vi "Modbus Status Interface.vi"(0 "ES System Data In":T8={"Voltage"=0.0, "Current"=0.0, "SOC Avg"=0.0, "Faults"=0, "Alarms"=0, "# Strings"=0, "Max Temp"=0, "Min Temp"=0, "Max Cell Voltage"=0.0, "Min Cell Voltage"=0.0, "Energy Capacity"=0.0, "Energy Remaining"=0.0, "SOC Min"=0.0, "SOC Max"=0.0, "ES Fault"=FALSE, "String Select"=enum."3 Strings", "ES Com Fault"=FALSE, "SOH Avg"=0.0}, 1 "ES String Data":T2, 2 "Gen Data Array":T4[](array[typedef]) {"TotalFuel(L)" format="%.2f"; "FuelRate(L/H)" format="%.2f"; "ApparentPower(VA)" format="%.2f"; "BattVoltage(V)" format="%.2f"; "Freq(Hz)" format="%.2f"; "RunHours(hr)" format="%.2f"; "PowerFactor" format="%.2f"; "ReactivePower(VAR)" format="%.2f"; "ActivePower(W)" format="%.2f"}, 3 "ES # Cycle Count":dbl, 5 "PC Data In":T6 {"Alarms 2" format="%016b"; "Faults 2" format="%016b"; "Alarms 1" format="%016b"; "Faults 1" format="%016b"; "Contactor FB" format="%.0b"; "DC Voltage SP" format="%2.1f"; "Clear Faults SP" format="%.0b"; "Neutral Current" format="%2.1f"; "AC Current - L2" format="%2.1f"; "AC Voltage - L2" format="%2.1f"; "Temperature" format="%2.1f"; "DC Voltage" format="%2.1f"; "AC Current SP" format="%2.1f"; "AC Voltage SP" format="%2.1f"; "Frequency SP" format="%2.1f"; "AC Frequency" format="%2.1f"; "AC Current - L1" format="%2.1f"; "AC Voltage- L1" format="%2.1f"}, 7 "isGenOn":bool[](array[boolean]), 9 "FPGA Data In":T5 {"SSG Active Current" format="%2.1f"; "PV Reactive Power (L1)" format="%2.1f"; "PV Reactive Power (L2)" format="%2.1f"; "PV Total Reactive Power" format="%2.1f"; "Gen Reactive Power (L1)" format="%2.1f"; "Gen Reactive Power (L2)" format="%2.1f"; "Gen Total Reactive Power" format="%2.1f"; "SSG Reactive Power (L1)" format="%2.1f"; "SSG Reactive Power (L2)" format="%2.1f"; "SSG Total Reactive Power" format="%2.1f"; "PV Total Current" format="%2.1f"; "PV Total Voltage" format="%2.1f"; "PV Active Power (L1)" format="%2.1f"; "PV Active Power (L2)" format="%2.1f"; "PV App Power (L1)" format="%2.1f"; "PV App Power (L2)" format="%2.1f"; "PV Total Active Power" format="%2.1f"; "PV Total App Power" format="%2.1f"; "PV Arms (L1)" format="%2.1f"; "PV Arms (L2)" format="%2.1f"; "PV Vrms (L1)" format="%2.1f"; "PV Vrms (L2)" format="%2.1f"; "Gen Total Current" format="%2.1f"; "SSG Total Current" format="%2.1f"; "Gen Total Voltage" format="%2.1f"; "SSG Total Voltage" format="%2.1f"; "Gen Active Power (L1)" format="%2.1f"; "Gen Active Power (L2)" format="%2.1f"; "SSG Active Power (L1)" format="%2.1f"; "SSG Active Power (L2)" format="%2.1f"; "Gen App Power (L1)" format="%2.1f"; "Gen App Power (L2)" format="%2.1f"; "SSG App Power (L1)" format="%2.1f"; "SSG App Power (L2)" format="%2.1f"; "Gen Total Active Power" format="%2.1f"; "Gen Total App Power" format="%2.1f"; "Gen Arms (L1)" format="%2.1f"; "Gen Arms (L2)" format="%2.1f"; "Gen Vrms (L1)" format="%2.1f"; "Gen Vrms (L2)" format="%2.1f"; "SSG Total Active Power" format="%2.1f"; "SSG Total App Power" format="%2.1f"; "SSG Arms (L1)" format="%2.1f"; "SSG Arms (L2)" format="%2.1f"; "SSG Vrms (L1)" format="%2.1f"; "SSG Vrms (L2)" format="%2.1f"}, 11 "Error In":errorcluster, 12 "Real Time State":T1) -> (15 "Error Out":errorcluster)   [LabVIEW 2014]
uses:
  Controls/ES System Data.ctl
  Controls/StringSelector.ctl
  Controls/PC Data.ctl
  Controls/MicroZed Config Op Mode.ctl
  Controls/FPGA Data.ctl
  Controls/Gen Data.ctl
  Controls/ES String Array.ctl
  Controls/ES String Data.ctl
  Controls/RT State.ctl
  Controls/Interface Data.ctl
panel:
  # "West"
  # "East"
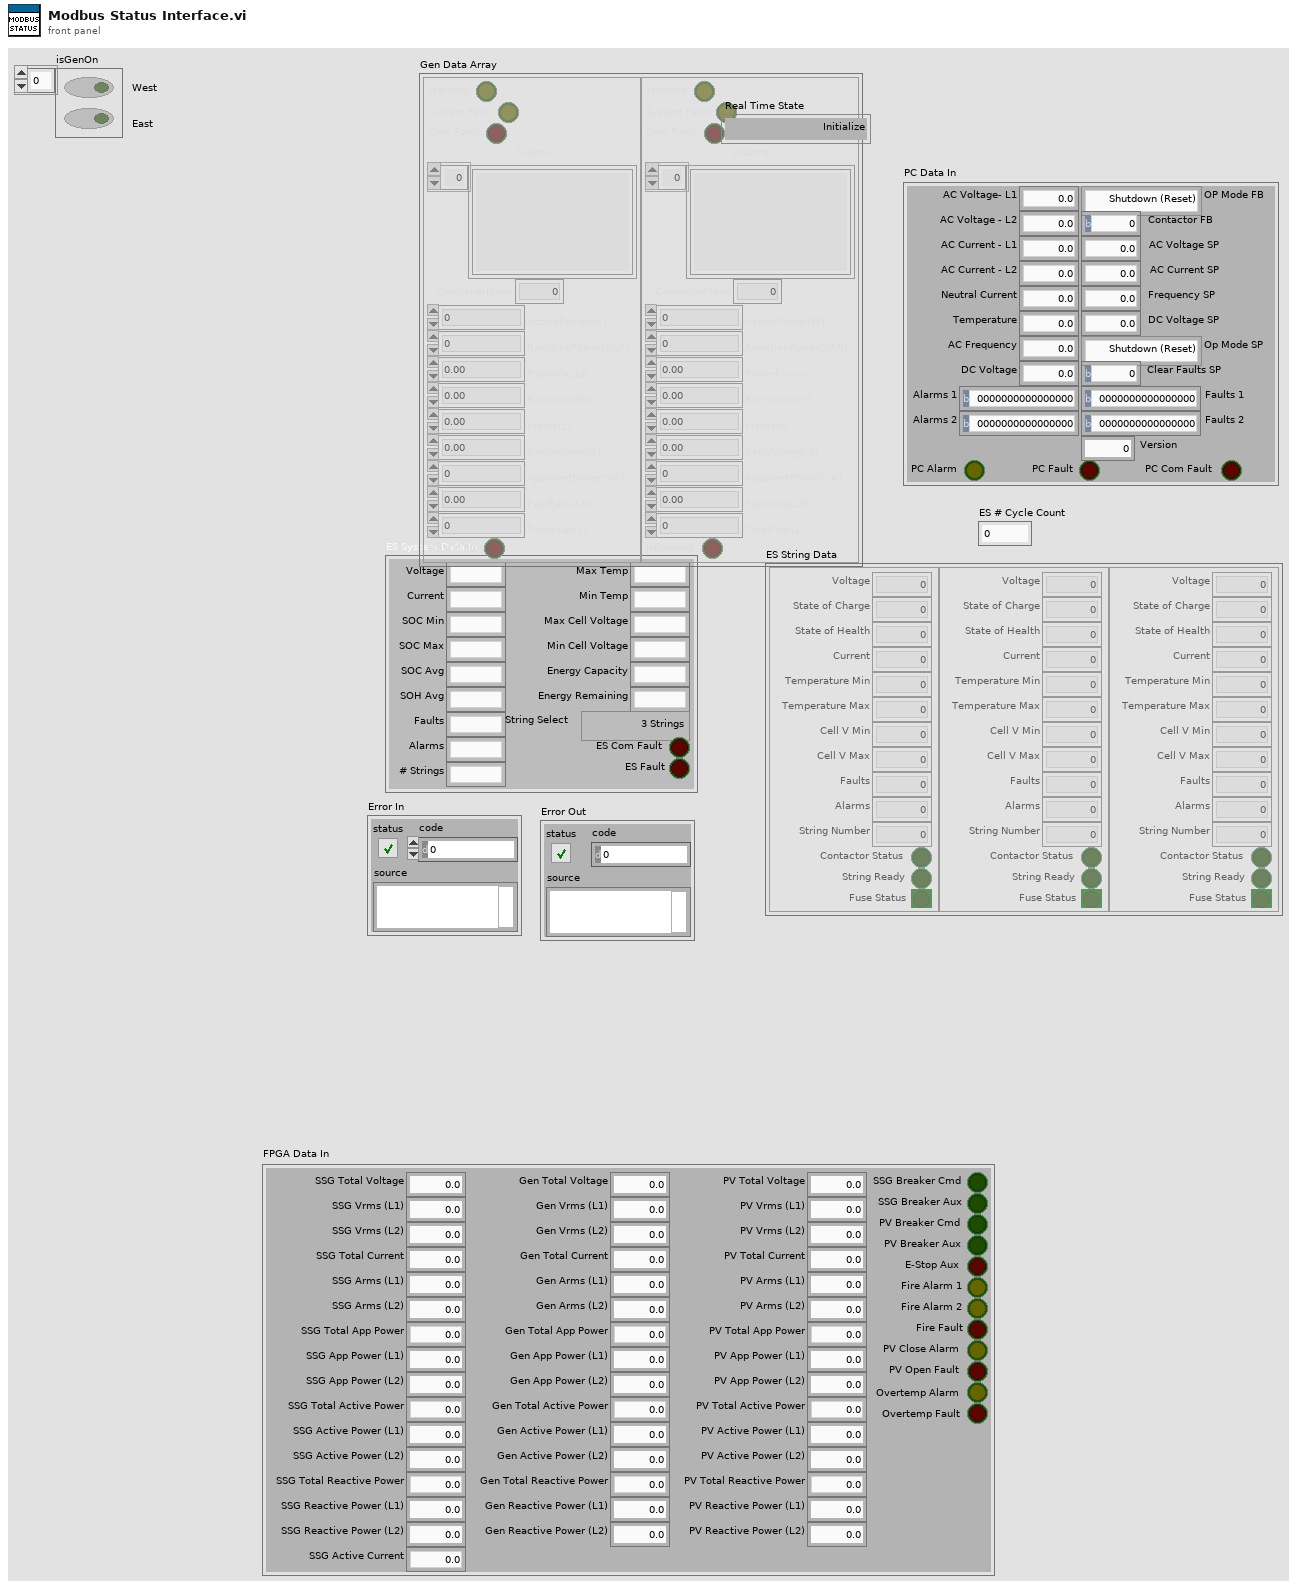
[diagram p1: front panel]
types:
  T1 = typedef "RT State.ctl" = enum16{"Initialize", "Ready", "Startup 1 - Start Genset", "Startup 2 - Start Inverter", "Startup 3 - Battery Match", "SpotGen - Start", "SpotGen - Charge", "SpotGen - Desync", "SpotGen - Discharge", "SpotGen - Sync", "Shutdown", "INVALID STATE"}
  T2 = typedef "ES String Array.ctl" = T3[]
  T3 = typedef "ES String Data.ctl" = cluster{"Voltage":sgl, "State of Charge":sgl, "Current":sgl, "Temperature Min":i16, "Temperature Max":i16, "Faults":u16, "Alarms":u16, "String Number":u16, "Contactor Status":bool, "String Ready":bool, "Fuse Status":bool, "Cell V Max":dbl, "Cell V Min":dbl, "State of Health":sgl}
  T4 = typedef "Gen Data.ctl" = cluster{"Warning":bool, "System Fault":bool, "Com Fault":bool, "Alarms":string[], "ControllerMode":u16, "ActivePower(W)":i32, "ReactivePower(VAR)":i32, "PowerFactor":dbl, "RunHours(hr)":dbl, "Freq(Hz)":dbl, "BattVoltage(V)":dbl, "ApparentPower(VA)":i32, "FuelRate(L/H)":dbl, "TotalFuel(L)":u32, "IsRunning":bool}
  T5 = typedef "FPGA Data.ctl" = cluster{"Gen Total Voltage":dbl, "Gen Vrms (L1)":dbl, "Gen Vrms (L2)":dbl, "Gen Total Current":dbl, "Gen Arms (L1)":dbl, "Gen Arms (L2)":dbl, "Gen Total App Power":dbl, "Gen App Power (L1)":dbl, "Gen App Power (L2)":dbl, "Gen Total Active Power":dbl, "Gen Active Power (L1)":dbl, "Gen Active Power (L2)":dbl, "Gen Total Reactive Power":dbl, "Gen Reactive Power (L1)":dbl, "Gen Reactive Power (L2)":dbl, "SSG Total Voltage":dbl, "SSG Vrms (L1)":dbl, "SSG Vrms (L2)":dbl, "SSG Total Current":dbl, "SSG Arms (L1)":dbl, "SSG Arms (L2)":dbl, "SSG Total App Power":dbl, "SSG App Power (L1)":dbl, "SSG App Power (L2)":dbl, "SSG Total Active Power":dbl, "SSG Active Power (L1)":dbl, "SSG Active Power (L2)":dbl, "SSG Total Reactive Power":dbl, "SSG Reactive Power (L1)":dbl, "SSG Reactive Power (L2)":dbl, "PV Total Voltage":dbl, "PV Vrms (L1)":dbl, "PV Vrms (L2)":dbl, "PV Total Current":dbl, "PV Arms (L1)":dbl, "PV Arms (L2)":dbl, "PV Total App Power":dbl, "PV App Power (L1)":dbl, "PV App Power (L2)":dbl, "PV Total Active Power":dbl, "PV Active Power (L1)":dbl, "PV Active Power (L2)":dbl, "PV Total Reactive Power":dbl, "PV Reactive Power (L1)":dbl, "PV Reactive Power (L2)":dbl, "SSG Breaker Cmd":bool, "SSG Breaker Aux":bool, "PV Breaker Cmd":bool, "PV Breaker Aux":bool, "E-Stop Aux":bool, "Fire Alarm 1":bool, "Fire Alarm 2":bool, "Fire Fault":bool, "PV Close Alarm":bool, "SSG Active Current":dbl, "Overtemp Alarm":bool, "Overtemp Fault":bool, "PV Open Fault":bool}
  T6 = typedef "PC Data.ctl" = cluster{"AC Voltage- L1":dbl, "AC Voltage - L2":dbl, "AC Current - L1":dbl, "AC Current - L2":dbl, "Neutral Current":dbl, "Temperature":dbl, "AC Frequency":dbl, "DC Voltage":dbl, "AC Voltage SP":dbl, "AC Current SP":dbl, "Frequency SP":dbl, "Op Mode SP":T7, "Clear Faults SP":u16, "PC Com Fault":bool, "PC Fault":bool, "DC Voltage SP":dbl, "OP Mode FB":T7, "Contactor FB":u16, "Faults 1":u16, "Alarms 1":u16, "Faults 2":u16, "Alarms 2":u16, "PC Alarm":bool, "Version":u16}
  T7 = typedef "MicroZed Config Op Mode.ctl" = enum16{"Shutdown (Reset)", "Startup", "Idle", "Voltage Mode", "Current Mode", "Fault", "OL Voltage (Debug)", "No Data"}
  T8 = typedef "ES System Data.ctl" = cluster{"Voltage":sgl, "Current":sgl, "SOC Avg":sgl, "Faults":u16, "Alarms":u16, "# Strings":u16, "Max Temp":i16, "Min Temp":i16, "Max Cell Voltage":sgl, "Min Cell Voltage":sgl, "Energy Capacity":sgl, "Energy Remaining":sgl, "SOC Min":sgl, "SOC Max":sgl, "ES Fault":bool, "String Select":T9, "ES Com Fault":bool, "SOH Avg":sgl}
  T9 = typedef "StringSelector.ctl" = enum16{"1 String (1)", "1 String (2)", "1 String (3)", "2 Strings (1 2)", "2 Strings (2 3)", "2 Strings (1 3)", "3 Strings"}
  T10 = typedef "Interface Data.ctl" = cluster{"SSG AC Current":i16, "SSG AC Voltage":i16, "SSC Active Power":i16, "SSG Reactive Power":i16, "SSG Apparent Power":i16, "SSG Frequency":i16, "ES SOC":i16, "ES SOH":i16, "ES Voltage":i16, "ES # Strings":i16, "ES # Cycles":i16, "ES Temperature":i16, "PC Temperature":i16, "Solar Active Power":i16, "Converter Version":i16, "Controller Version":i16, "System Status":i16, "System Faults":i16, "Controller Faults":i16, "ES System Faults":i16, "ES System Alarms":i16, "Converter Faults 1":i16, "Converter Faults 2":i16, "Converter Alarms 1":i16, "Converter Alarms 2":i16, "Solar Faults":i16, "ES Rack 1 Faults":i16, "ES Rack 2 Faults":i16, "ES Rack 3 Faults":i16, "ES Rack 4 Faults":i16, "ES Rack 5 Faults":i16, "ES Rack 6 Faults":i16, "ES Rack 7  Faults":i16, "ES Rack 8 Faults":i16, "ES Rack 9 Faults":i16, "ES Rack 10 Faults":i16, "ES Rack 1 Alarms":i16, "ES Rack 2 Alarms":i16, "ES Rack 3 Alarms":i16, "ES Rack 4 Alarms":i16, "ES Rack 5 Alarms":i16, "ES Rack 6 Alarms":i16, "ES Rack 7 Alarms":i16, "ES Rack 8 Alarms":i16, "ES Rack 9 Alarms":i16, "ES Rack 10 Alarms":i16, "GenWest":T4, "GenEast":T4}
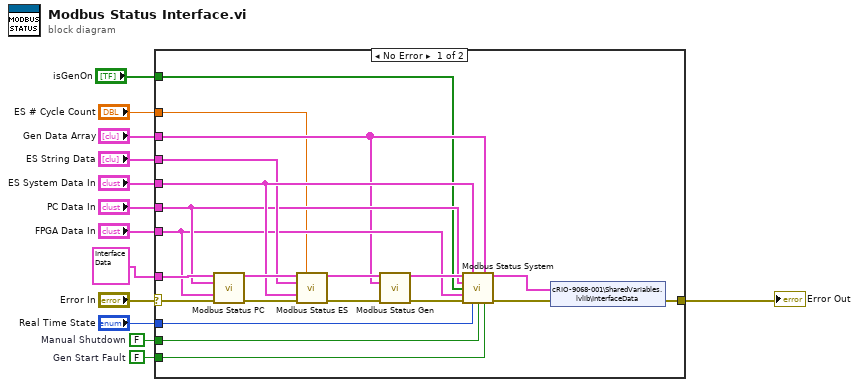
[diagram p0: block diagram]
diagram:
  w4 = FALSE  # Manual Shutdown
  w3 = FALSE  # Gen Start Fault
  n1 = case shown="No Error" "Error In" {
    selector: "Error In" -> [w34 w35]
    tunnel: [w14 w35] -> w12
    tunnel: "FPGA Data In" -> [w23 _]
    tunnel: "PC Data In" -> [w24 _]
    tunnel: "ES System Data In" -> [w26 _]
    tunnel: "Gen Data Array" -> [w21 _]
    tunnel: T10 {"SSG AC Current"=0, "SSG AC Voltage"=0, "SSC Active Power"=0, "SSG Reactive Power"=0, "SSG Apparent Power"=0, "SSG Frequency"=0, "ES SOC"=0, "ES SOH"=0, "ES Voltage"=0, "ES # Strings"=0, "ES # Cycles"=0, "ES Temperature"=0, "PC Temperature"=0, "Solar Active Power"=0, "Converter Version"=0, "Controller Version"=0, "System Status"=0, "System Faults"=0, "Controller Faults"=0, "ES System Faults"=0, "ES System Alarms"=0, "Converter Faults 1"=0, "Converter Faults 2"=0, "Converter Alarms 1"=0, "Converter Alarms 2"=0, "Solar Faults"=0, "ES Rack 1 Faults"=0, "ES Rack 2 Faults"=0, "ES Rack 3 Faults"=0, "ES Rack 4 Faults"=0, "ES Rack 5 Faults"=0, "ES Rack 6 Faults"=0, "ES Rack 7  Faults"=0, "ES Rack 8 Faults"=0, "ES Rack 9 Faults"=0, "ES Rack 10 Faults"=0, "ES Rack 1 Alarms"=0, "ES Rack 2 Alarms"=0, "ES Rack 3 Alarms"=0, "ES Rack 4 Alarms"=0, "ES Rack 5 Alarms"=0, "ES Rack 6 Alarms"=0, "ES Rack 7 Alarms"=0, "ES Rack 8 Alarms"=0, "ES Rack 9 Alarms"=0, "ES Rack 10 Alarms"=0, "GenWest"={"Warning"=FALSE, "System Fault"=FALSE, "Com Fault"=FALSE, "Alarms"=[], "ControllerMode"=0, "ActivePower(W)"=0, "ReactivePower(VAR)"=0, "PowerFactor"=0.0, "RunHours(hr)"=0.0, "Freq(Hz)"=0.0, "BattVoltage(V)"=0.0, "ApparentPower(VA)"=0, "FuelRate(L/H)"=0.0, "TotalFuel(L)"=0, "IsRunning"=FALSE}, "GenEast"={"Warning"=FALSE, "System Fault"=FALSE, "Com Fault"=FALSE, "Alarms"=[], "ControllerMode"=0, "ActivePower(W)"=0, "ReactivePower(VAR)"=0, "PowerFactor"=0.0, "RunHours(hr)"=0.0, "Freq(Hz)"=0.0, "BattVoltage(V)"=0.0, "ApparentPower(VA)"=0, "FuelRate(L/H)"=0.0, "TotalFuel(L)"=0, "IsRunning"=FALSE}} ("Modbus Status Interface Data In") -> [w29 _]
    tunnel: "ES String Data" -> [w25 _]
    tunnel: "Real Time State" -> [w22 _]
    tunnel: w4 -> [w20 _]
    tunnel: w3 -> [w19 _]
    tunnel: "ES # Cycle Count" -> [w18 _]
    tunnel: "isGenOn" -> [w17 _]
    frame No Error {
      n2 = call "Modbus Status PC.vi"("InterfaceData"=w29, "PC Data In"=w24, "FPGA Data In"=w23, "Error In"=w34) -> ("InterfaceData"=w31:T10, "Error Out"=w33:errorcluster)  [unwired: 10 in]
      n3 = call "Modbus Status ES.vi"("InterfaceData"=w31, "ES Cycle Count"=w18, "ES String Data"=w25, "ES System Data In"=w26, "Error In"=w33) -> ("InterfaceData"=w30:T10, "Error Out"=w32:errorcluster)  [unwired: 9 in]
      n4 = call "Modbus Status Gen.vi"("InterfaceData"=w30, "Gen Data Array"=w21, "Error In"=w32) -> ("InterfaceData"=w27:T10, "Error Out"=w28:errorcluster)  [unwired: 11 in]
      n5 = call "Modbus Status System.vi"("InterfaceData"=w27, "ES System Data In"=w26, "Gen Data Array"=w21, "PC Data In"=w24, "isGenOn"=w17, "FPGA Data In"=w23, "Error In"=w28, "Real Time State"=w22, "Manual Shutdown"=w20, "Gen Start Fault"=w19) -> ("InterfaceData"=w16:T10, "Error Out"=w15:errorcluster)  [unwired: 4 in]
      n6 = shared-variable "cRIO-9068-001\\SharedVariables.lvlib\\InterfaceData"(w16, error in=w15) -> (error out=w14:errorcluster)
    }
    frame Error {
    }
  }
  "Error Out" <- w12
